vi "LocalizationUnitTestSuite.vi"() -> ()   [LabVIEW 2017]
uses:
  <vilib>/addons/_JKI Toolkits/Caraya/classes/Test Suite/Test Suite.lvclass
panel:
  in  "Interactive":bool=TRUE
  in  "Report Path (leave blank if interactive = true)":path
  # "Run me to run all Localization unit tests"
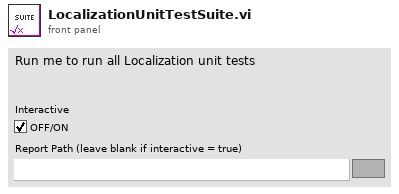
[diagram p1: front panel]
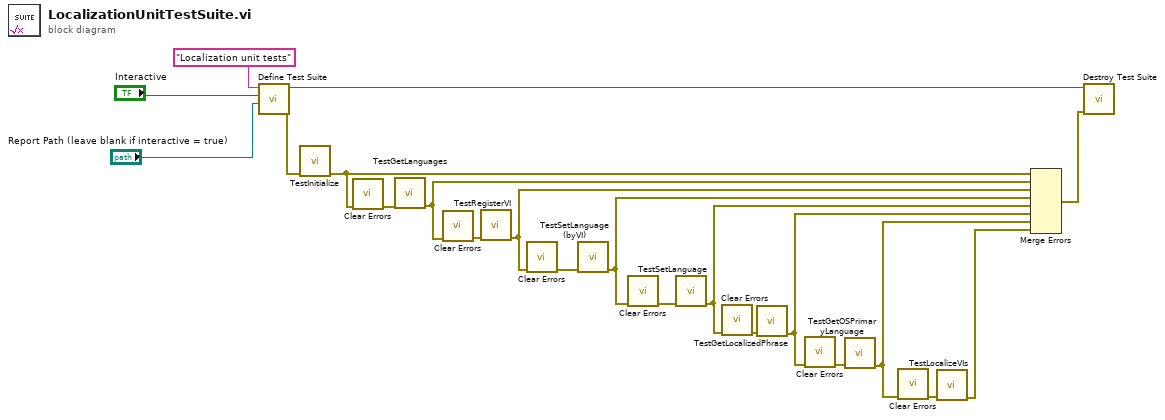
[diagram p0: block diagram]
diagram:
  n1 = call <vilib>:"Define Test Suite.vi"("Report Path"="Report Path (leave blank if interactive = true)", "Interactive"="Interactive", "Label (VI Title)"="Localization unit tests") -> ("error out"=w18:errorcluster, "Test Suite"=w17:refnum<class "Test Suite.lvclass">)  [unwired: 7 in]
  n2 = call "TestInitialize.vi"("error in (no error)"=w18) -> ("error out"=w15:errorcluster)  [unwired: 10 in]
  n3 = call <vilib>:"Clear Errors.vi"("error in (no error)"=w15) -> ("error out"=w16:errorcluster)  [unwired: 5 in, 1 out]
  n4 = call "TestGetLanguages.vi"("error in (no error)"=w16) -> ("error out"=w14:errorcluster)  [unwired: 10 in]
  n5 = call <vilib>:"Clear Errors.vi"("error in (no error)"=w14) -> ("error out"=w13:errorcluster)  [unwired: 5 in, 1 out]
  n6 = call "TestRegisterVI.vi"("error in (no error)"=w13) -> ("error out"=w11:errorcluster)  [unwired: 10 in]
  n7 = call <vilib>:"Clear Errors.vi"("error in (no error)"=w11) -> ("error out"=w12:errorcluster)  [unwired: 5 in, 1 out]
  n8 = call "TestSetLanguage(byVI).vi"("error in (no error)"=w12) -> ("error out"=w10:errorcluster)  [unwired: 10 in]
  n9 = call <vilib>:"Clear Errors.vi"("error in (no error)"=w10) -> ("error out"=w9:errorcluster)  [unwired: 5 in, 1 out]
  n10 = call "TestSetLanguage.vi"("error in (no error)"=w9) -> ("error out"=w7:errorcluster)  [unwired: 10 in]
  n11 = call <vilib>:"Clear Errors.vi"("error in (no error)"=w7) -> ("error out"=w8:errorcluster)  [unwired: 5 in, 1 out]
  n12 = call "TestGetLocalizedPhrase.vi"("error in (no error)"=w8) -> ("error out"=w5:errorcluster)  [unwired: 10 in]
  n13 = call <vilib>:"Clear Errors.vi"("error in (no error)"=w5) -> ("error out"=w6:errorcluster)  [unwired: 5 in, 1 out]
  n14 = call "TestGetOSPrimaryLanguage.vi"("error in (no error)"=w6) -> ("error out"=w3:errorcluster)  [unwired: 10 in]
  n15 = call <vilib>:"Clear Errors.vi"("error in (no error)"=w3) -> ("error out"=w4:errorcluster)  [unwired: 5 in, 1 out]
  n16 = call "TestLocalizeVIs.vi"("error in (no error)"=w4) -> ("error out"=w2:errorcluster)  [unwired: 10 in]
  n17 = Merge Errors(w15, w14, w11, w10, w7, w5, w3, w2) -> (w1:errorcluster)
  n18 = call-dynamic "Destroy Test Suite.vi"("error in (no error)"=w1, "Test Suite in"=w17) -> ()  [unwired: 9 in, 1 out]
